vi "MVE Get TDs.vi"(7 "error in (no error)":errorcluster) -> (0 "IDs":string[](array[string]), 1 "TD sizes":string[](array[string]), 2 "Typedescs":u8[](array[numeric]), 3 "names":string[](array[string]))   [LabVIEW 2016]
panel:
  out "size(s)":i32
  out "total size":i32
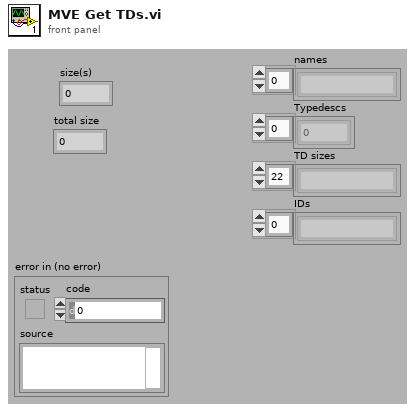
[diagram p1: front panel]
types:
  T1 = typedef "SCT Default Types.ctl" = cluster{"names":string[], "TDs":T2[]}
  T2 = typedef "NI_Variable.lvlib/Type Descriptor.ctl" = cluster{"Variant":variant}
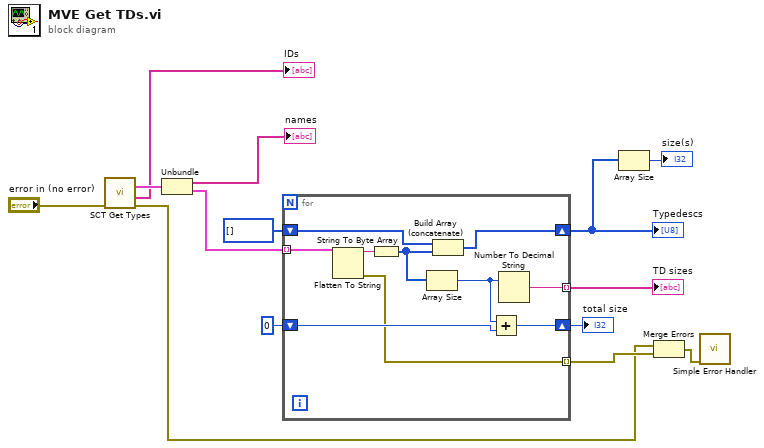
[diagram p0: block diagram]
diagram:
  n1 = call <resource>:"SCT Get Types.vi"("error in"="error in (no error)") -> ("error out"=w4:errorcluster, "IDs"=→"IDs":string[], "default types"=w14:T1)  [unwired: 8 in]
  n2 = Unbundle(w14) -> ("names"=→"names":string[], "TDs"=w12:T2[])
  n3 = for {
    tunnel: w12 -> [w24] mode=indexing
    shift-right: [w22] -> w9
    shift-left: u8[] [] ("unsigned byte array") -> [w21]
    tunnel: [w19] -> w10 mode=indexing
    shift-right: [w17] -> w7
    shift-left: 0 -> [w16]
    tunnel: [w15] -> w5 mode=indexing
    n4 = Flatten To String(anything=w24) -> (data string=w23:string, error out=w15:errorcluster)  [unwired: 3 in, 1 out]
    n5 = String To Byte Array(string=w23) -> (unsigned byte array=w20:u8[])
    n6 = Array Size(array=w20) -> (size(s)=w18:i32)
    n7 = Build Array (concatenate)(w21, w20) -> (w22:u8[])
    n8 = Add(x=w18, y=w16) -> (x+y=w17:i32)
    n9 = Number To Decimal String(number=w18) -> (decimal integer string=w19:string)  [unwired: 1 in]
  }
  "Typedescs" <- w9
  "TD sizes" <- w10
  "total size" <- w7
  n10 = Array Size(array=w9) -> (size(s)=→"size(s)":i32)
  n11 = Merge Errors(w4, w5) -> (w2:errorcluster)
  n12 = call <vilib>:"Simple Error Handler.vi"("error in (no error)"=w2) -> ()  [unwired: 4 in, 5 out]
